vi "3D vector length.vi"(8 "Pos/Vel":enum16{"Position", "Velocity"}(ring)=enum."Velocity", 9 "Eye":enum16{"Right", "Left"}(ring), 10 "Channel Groups":i32[][][](array[numeric]), 11 "Data Channels in":dbl[][](array[numeric])) -> (3 "Data Channels out":dbl[](array[numeric]))   [LabVIEW 2016]
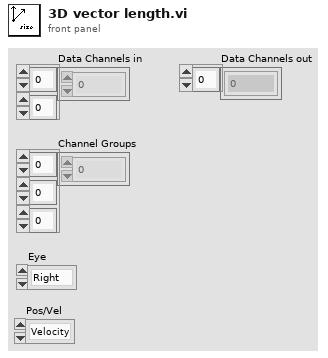
[diagram p1: front panel]
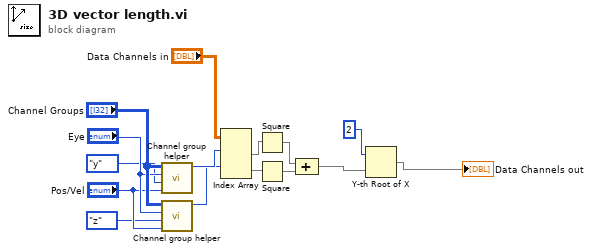
[diagram p0: block diagram]
diagram:
  n1 = call "Channel group helper.vi"("Pos/Vel"="Pos/Vel", "Eye component"=enum16{"x", "y", "z"}."y", "Eye"="Eye", "Channel Groups"="Channel Groups") -> ("Channel"=w2:i32)  [unwired: 7 in]
  n2 = call "Channel group helper.vi"("Pos/Vel"="Pos/Vel", "Eye component"=enum16{"x", "y", "z"}."z", "Eye"="Eye", "Channel Groups"="Channel Groups") -> ("Channel"=w1:i32)  [unwired: 7 in]
  n3 = Index Array(array="Data Channels in", index (row) #1=w2, index (row) #2=w1) -> (element #1=w9:dbl[], element #2=w8:dbl[])  [unwired: 2 in]
  n4 = Square(x=w9) -> (x^2=w7:dbl[])
  n5 = Square(x=w8) -> (x^2=w6:dbl[])
  n6 = Compound Arithmetic op=ADD(w7, w6) -> (w5:dbl[])
  n7 = Y-th Root of X(1:w5, 2:2) -> (0:→"Data Channels out":dbl[])
